vi "csmdoc_import_doc_to_singleVI.vi"() -> ()   [LabVIEW 2017, in "csmdoc.lvlib"]
uses:
  csmdoc.lvlib
panel:
  in  "VI":path=path "D:/CSM Framework/Communicable-State-Machine/src/user.lib/_NEVSTOP/Communicable State Machine(CSM)/Parse State Queue++.vi"
  in  "Error in":errorcluster caption="Error in (no error)"
  out "error out":errorcluster
  in  "doc":path=path "D:/CSM Framework/Communicable-State-Machine/src/help/NEVSTOP/Communicable State Machine(CSM)/VI Description(CN).md"
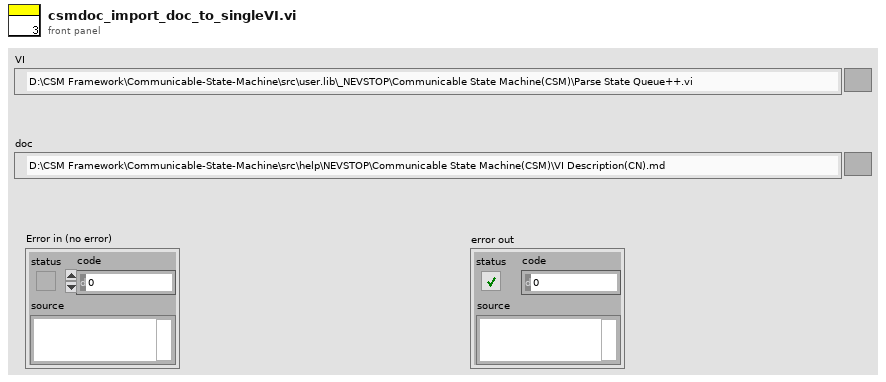
[diagram p1: front panel]
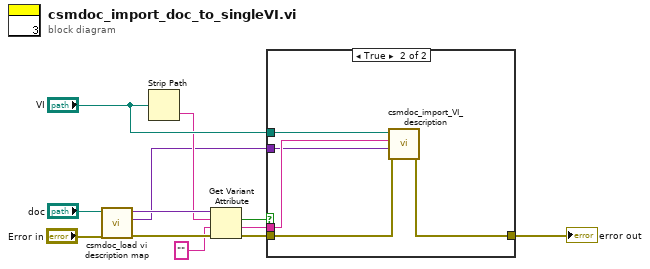
[diagram p0: block diagram]
diagram:
  n1 = call "csmdoc_load vi description map.vi"("Error in"="Error in", "Path"="doc") -> ("Error out"=w10:errorcluster, "variant 2"=w1:variant, "variant"=w12:variant)  [unwired: 6 in, 1 out]
  n2 = Strip Path(path="VI") -> (name=w6:string)  [unwired: 1 out]
  n3 = Get Variant Attribute(Variant=w12, name=w6, default value (empty Variant)="" ("String"), error in=w10) -> (found=w5:bool, value=w2:string, error out=w4:errorcluster)  [unwired: 1 out]
  n4 = case shown="True" w5 {
    tunnel: "VI" -> [_ w18]
    tunnel: w4 -> [w13 w17]
    tunnel: [w13 w16] -> w9
    tunnel: w2 -> [_ w15]
    tunnel: w1 -> [_ w14]
    frame False {
    }
    frame True {
      n5 = call "csmdoc_import_VI_description.vi"("error in (no error)"=w17, "NOTE-Map"=w14, "string"=w15, "Path"=w18) -> ("error out"=w16:errorcluster)  [unwired: 7 in]
    }
  }
  "error out" <- w9
